vi "WriteRate.vi"(8 "error in (no error)":errorcluster, 10 "Rate":dbl, 11 "DataVer1 in":refnum<class "DataVer1.lvclass">) -> (0 "error out":errorcluster, 3 "DataVer1 out":refnum<class "DataVer1.lvclass">)   [LabVIEW 2013, in "DataVer1.lvclass"]
uses:
  DataVer1.lvclass
  DataVer1.lvclass/DataVer1.ctl
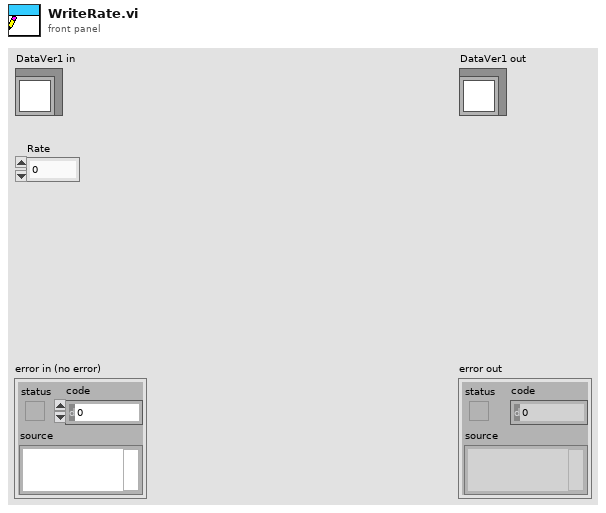
[diagram p1: front panel]
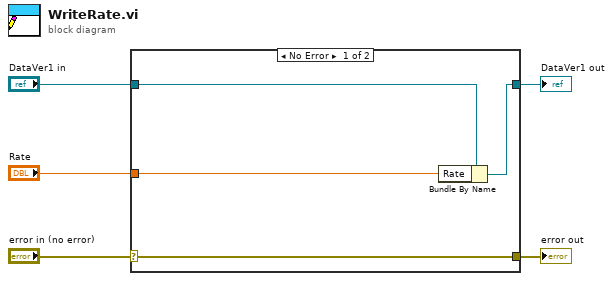
[diagram p0: block diagram]
diagram:
  n1 = case shown="No Error" "error in (no error)" {
    selector: "error in (no error)" -> [w9 w10]
    tunnel: [w9 w10] -> w4
    tunnel: [w7 w11] -> w2
    tunnel: "DataVer1 in" -> [w8 w11]
    tunnel: "Rate" -> [w6 _]
    frame No Error {
      n2 = Bundle By Name(cluster=w8, "Rate"=w6) -> (w7:refnum<class "DataVer1.lvclass">)
    }
    frame Error {
    }
  }
  "error out" <- w4
  "DataVer1 out" <- w2
